vi "DestroyPrivateEvents.vi"(8 "error in (no error)":errorcluster, 11 "EmbeddedSMO":refnum<class "Embedded UI.lvclass">) -> (0 "error out":errorcluster, 3 "EmbeddedSMO out":refnum<class "Embedded UI.lvclass">)   [LabVIEW 2019, in "Embedded UI.lvclass"]
doc: "JKI State Machine Objects (SMO) 1.0.0.5\nJKI - JKI\nCopyright (c) 2016, JKI"
uses:
  Embedded UI.lvclass
  <vilib>/JKI/JKI SMO/SMO.UI/SMO.UI.lvclass
panel:
  # "For instructions on how to use the JKI State Machine Objects, examples and video tutorials, visit:\nhttp://jki.net/state-machine-objects/\n\nJKI State Machine Objects™\nhttp://jki.net/state-machine-objects/\nCopyright (C) 2005-2015, JKI <info@jki.net>\nALL RIGHTS RESERVED"
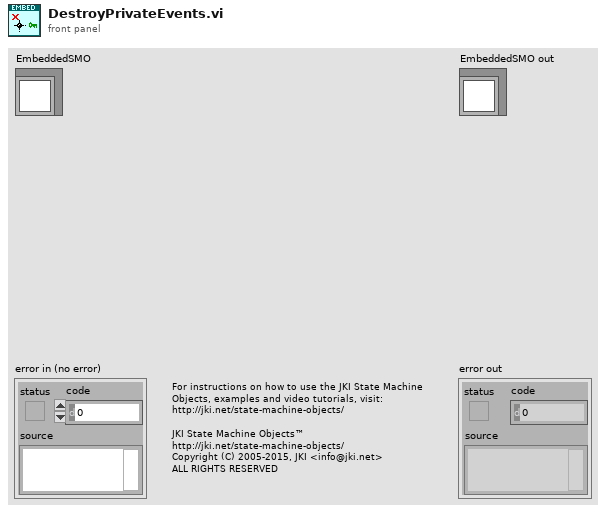
[diagram p1: front panel]
types:
  T1 = typedef "Embedded UI.lvclass/PrivateEvents--Cluster.ctl" = cluster{"Get UI State":refnum<user-event>, "SetUIState":refnum<user-event>, "GetSubPanelReference":refnum<user-event>, "SetSubpanelReference":refnum<user-event>, "WriteName":refnum<user-event>, "GetName":refnum<user-event>}
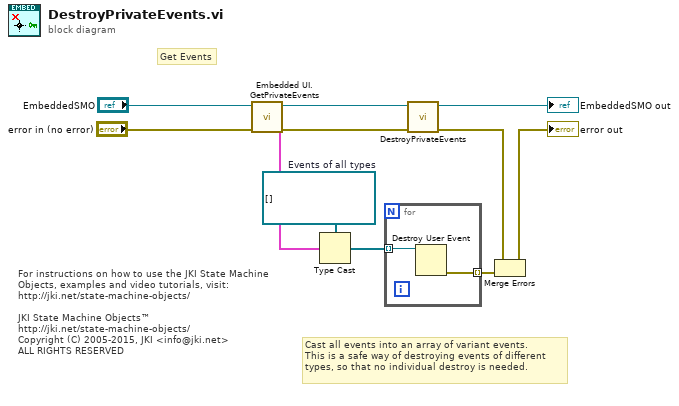
[diagram p0: block diagram]
diagram:
  w7 = refnum<user-event>[] []  # Events of all types
  # "Get Events"
  # "For instructions on how to use the JKI State Machine Objects, examples and video tutorials, visit:\nhttp://jki.net/state-machine-objects/\n\nJKI State Machine Objects™\nhttp://jki.net/state-machine-objects/\nCopyright (C) 2005-2015, JKI <info@jki.net>\nALL RIGHTS RESERVED"
  # "Cast all events into an array of variant events.\nThis is a safe way of destroying events of different\ntypes, so that no individual destroy is needed."
  n1 = call "Embedded UI.GetPrivateEvents.vi"("error in (no error)"="error in (no error)", "EmbeddedSMO"="EmbeddedSMO") -> ("error out"=w4:errorcluster, "Private Events"=w1:T1, "EmbeddedSMO out"=w3:refnum<class "Embedded UI.lvclass">)  [unwired: 7 in]
  n2 = Type Cast(type=w7, x=w1) -> (*(type *) &x=w8:refnum<user-event>[])
  n3 = for {
    tunnel: w8 -> [w13] mode=indexing
    tunnel: [w12] -> w6 mode=indexing
    n4 = Destroy User Event(user event=w13) -> (error out=w12:errorcluster)  [unwired: 1 in]
  }
  n5 = call-parent "DestroyPrivateEvents.vi"("error in (no error)"=w4, "SMO.UI"=w3) -> ("error out"=w10:errorcluster, "SMO.UI out"=→"EmbeddedSMO out":refnum<class "Embedded UI.lvclass">)  [unwired: 8 in]
  n6 = Merge Errors(w10, w6) -> (→"error out":errorcluster)
